vi "Standby.vi"(8 "error in (no error)":errorcluster, 10 "Model in":refnum<class "Model.lvclass">, 11 "Fault State in":refnum<class "Fault State.lvclass">) -> (0 "error out":errorcluster, 2 "Model out":refnum<class "Model.lvclass">, 3 "Fault State out":refnum<class "Fault State.lvclass">)   [LabVIEW 2016, in "Fault State.lvclass"]
uses:
  Fault State.lvclass
  Model/Model/Model.lvclass
  Typedefs/StateTypes.ctl
  Typedefs/HPMT_Typedefs.lvlib
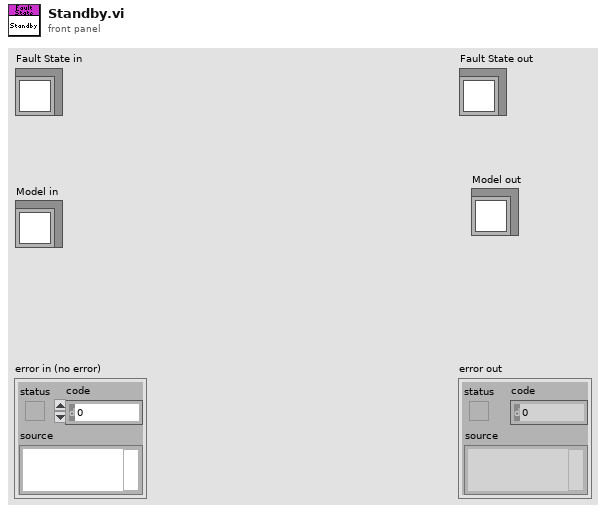
[diagram p1: front panel]
types:
  T1 = typedef "HPMT_Typedefs.lvlib/StateTypes.ctl" = enum16{"Offline State", "Fault State", "Standby State", "Disabled State", "Enabled State", "Wait For User Input State", "Test Actuator State"}
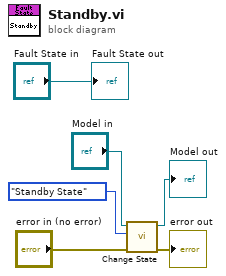
[diagram p0: block diagram]
diagram:
  n1 = call "Change State.vi"("error in (no error)"="error in (no error)", "State Types"=StateTypes."Standby State" ("State:"), "Model in"="Model in") -> ("error out"=→"error out":errorcluster, "Model out"=→"Model out":refnum<class "Model.lvclass">)  [unwired: 7 in]
  "Fault State out" <- "Fault State in"
